vi "ControlReference.CreateReferenceToControls.vi"(8 "error in (no error)":errorcluster, 11 "pathToMainVI":path) -> (0 "error out":errorcluster, 3 "referenceToControls":refnum<vi>[](array[refnum]))   [LabVIEW 2019]
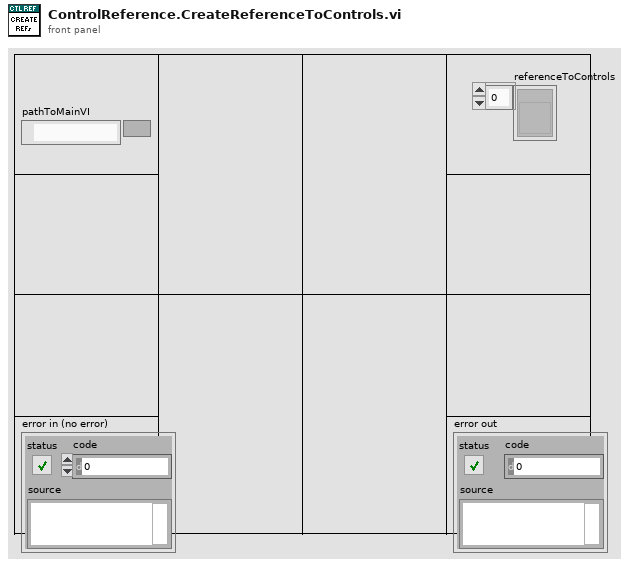
[diagram p1: front panel]
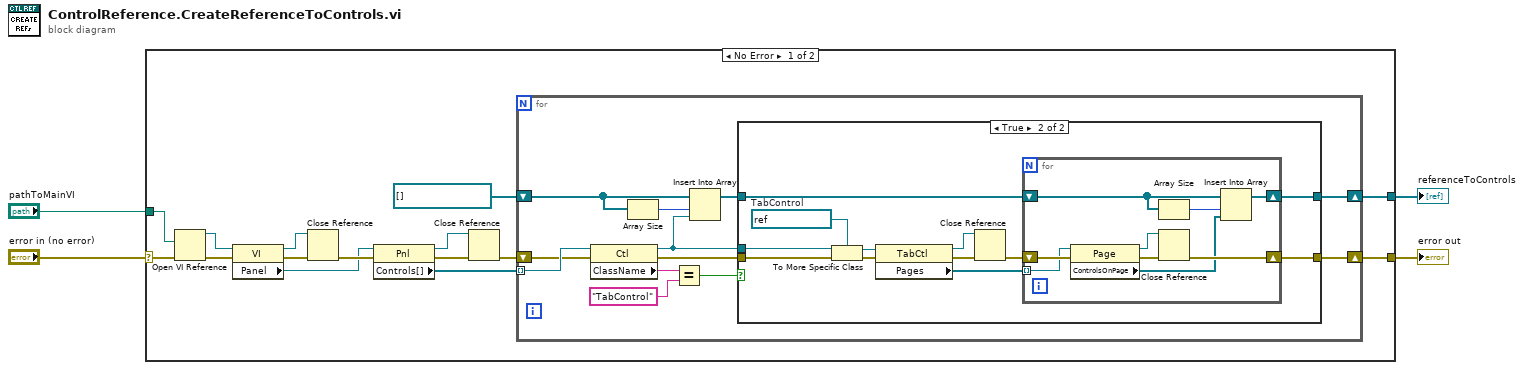
[diagram p0: block diagram]
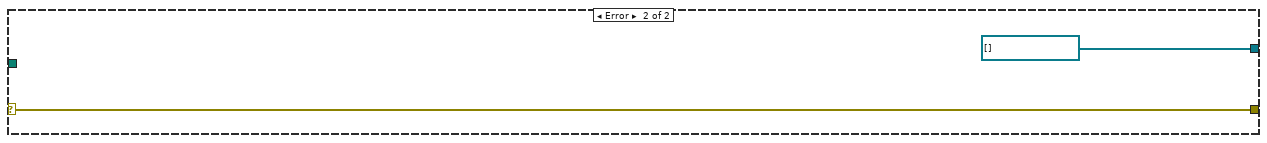
[diagram p3: hidden frame]
diagram:
  n1 = case shown="No Error" "error in (no error)" {
    selector: "error in (no error)" -> [w7 w56]
    tunnel: [w11 w56] -> w3
    tunnel: [w9 refnum<vi>[] []] -> w4
    tunnel: "pathToMainVI" -> [w8 _]
    frame No Error {
      n2 = Open VI Reference(vi path=w8, error in (no error)=w7) -> (vi reference=w5:refnum<vi>, error out=w6:errorcluster)  [unwired: 4 in]
      n3 = property class="VI"(reference=w5, error in=w6) -> (reference out=w18:refnum<vi>, error out=w19:errorcluster, "Panel"=w16:refnum<vi>)
      n4 = Close Reference(reference=w18, error in (no error)=w19) -> (error out=w17:errorcluster)
      n5 = property class="Pnl"(reference=w16, error in=w17) -> (reference out=w14:refnum<vi>, error out=w13:errorcluster, "Controls[]"=w15:refnum<vi>[])
      n6 = Close Reference(reference=w14, error in (no error)=w13) -> (error out=w12:errorcluster)
      n7 = for {
        shift-right: [w27] -> w11
        shift-left: w12 -> [w30]
        tunnel: w15 -> [w31] mode=indexing
        shift-right: [w25] -> w9
        shift-left: refnum<vi>[] [] -> [w24]
        n8 = property class="Ctl"(reference=w31, error in=w30) -> (reference out=w21:refnum<vi>, error out=w20:errorcluster, "ClassName"=w29:string)
        n9 = Array Size(array=w24) -> (size(s)=w22:i32)
        n10 = Equal?(x=w29, y="TabControl") -> (x = y?=w26:bool)
        n11 = Insert Into Array(array=w24, index=w22, new element=w21) -> (w23:refnum<vi>[])
        n12 = case shown="True" w26 {
          tunnel: [w33 w37] -> w27
          tunnel: w20 -> [w33 w44]
          tunnel: w21 -> [_ w45]
          tunnel: [w32 w35] -> w25
          tunnel: w23 -> [w32 w34]
          frame False {
          }
          frame True {
            w42 = refnum<vi> refnum  # TabControl
            n13 = To More Specific Class(target class=w42, reference=w45, error in=w44) -> (specific class reference=w41:refnum<vi>, error out=w43:errorcluster)
            n14 = property class="TabCtl"(reference=w41, error in=w43) -> (reference out=w40:refnum<vi>, error out=w39:errorcluster, "Pages"=w36:refnum<vi>[])
            n15 = Close Reference(reference=w40, error in (no error)=w39) -> (error out=w38:errorcluster)
            n16 = for {
              shift-right: [w51] -> w37
              shift-left: w38 -> [w54]
              tunnel: w36 -> [w53] mode=indexing
              shift-right: [w48] -> w35
              shift-left: w34 -> [w46]
              n17 = property class="Page"(reference=w53, error in=w54) -> (reference out=w50:refnum<vi>, error out=w52:errorcluster, "ControlsOnPage"=w49:refnum<vi>[])
              n18 = Array Size(array=w46) -> (size(s)=w47:i32)
              n19 = Close Reference(reference=w50, error in (no error)=w52) -> (error out=w51:errorcluster)
              n20 = Insert Into Array(array=w46, index=w47, new element=w49) -> (w48:refnum<vi>[])
            }
          }
        }
      }
    }
    frame Error {
    }
  }
  "referenceToControls" <- w4
  "error out" <- w3
